vi "vision0.vi"(0 "Color Plane (Color Plane Extraction 1)":i32(ring)=2 items=["Red", "Green", "Blue", "Hue", "Saturation", "Luminance", "Value", "Intensity"], 1 "Range (Threshold 1)":cluster{"Lower value":sgl, "Upper value":sgl}={"Lower value"=199.0, "Upper value"=255.0}, 2 "Number of Erosion (Adv. Morphology 1)":i32=1, 3 "Square/Hexa (Square) (Adv. Morphology 1)":bool, 4 "Connectivity 4/8 (8) (Adv. Morphology 1)":bool=TRUE, 5 "Low Pass/High Pass (Low) (Adv. Morphology 1)":bool, 7 "error in":errorcluster) -> (20 "Number of Matches (Shape Matching 1)":i32, 21 "Shape Report (calibrated) (Shape Matching 1)":T2(array[cluster]) {"Score" format="%.2f"; "Centroid"."y" format="%.2f"; "Centroid"."x" format="%.2f"}, 22 "Centroid (Centroid 1)":cluster{"X Centroid":sgl, "Y Centroid":sgl} {"Y Centroid" format="%.2f"; "X Centroid" format="%.2f"}, 23 "Calibrated Centroid (Centroid 1)":cluster{"X Centroid":sgl, "Y Centroid":sgl} {"Y Centroid" format="%.2f"; "X Centroid" format="%.2f"}, 27 "error out":errorcluster)   [LabVIEW 2016]
uses:
  <vilib>/vision/NI_Vision_Development_Module.lvlib
panel:
  out "Image Out":T1(plugin-control)
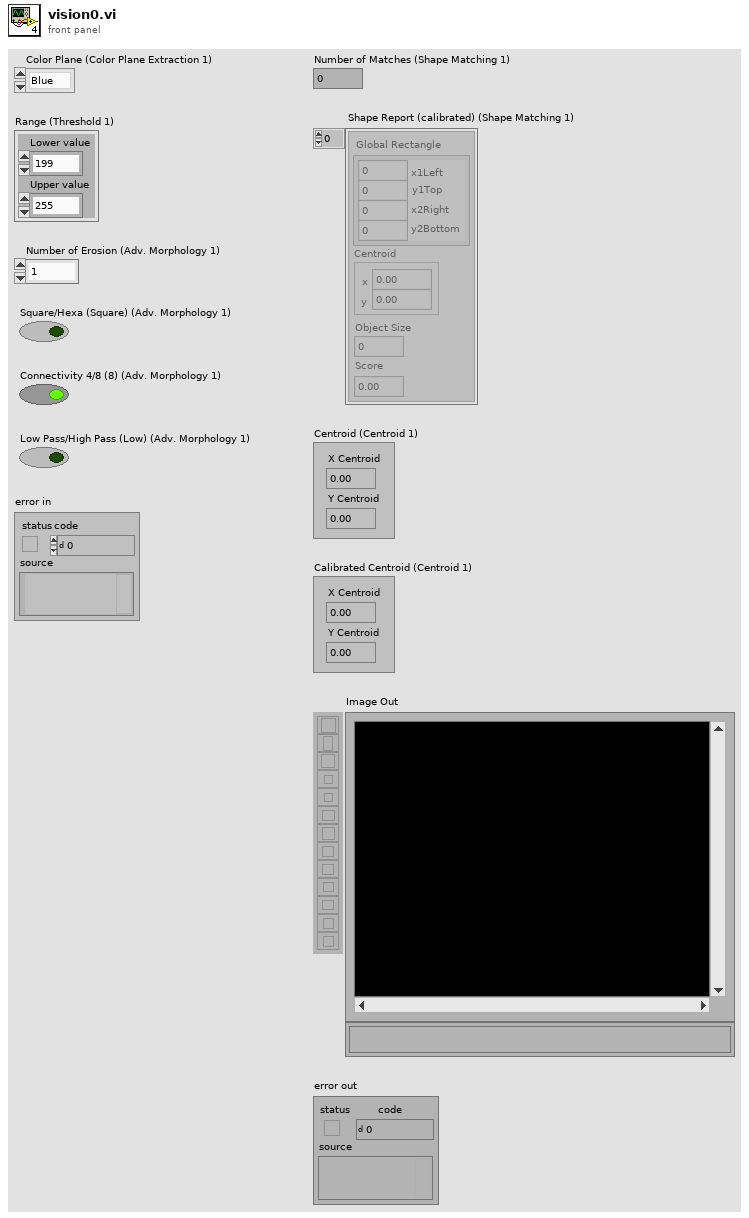
[diagram p1: front panel]
types:
  T1 = typedef "IMAQ Image.ctl" = refnum<image>
  T2 = cluster{"Global Rectangle":cluster{"x1Left":i32, "y1Top":i32, "x2Right":i32, "y2Bottom":i32}, "Centroid":cluster{"x":sgl, "y":sgl}, "Object Size":u32, "Score":dbl}[]
  T3 = typedef "Image Type" = u32
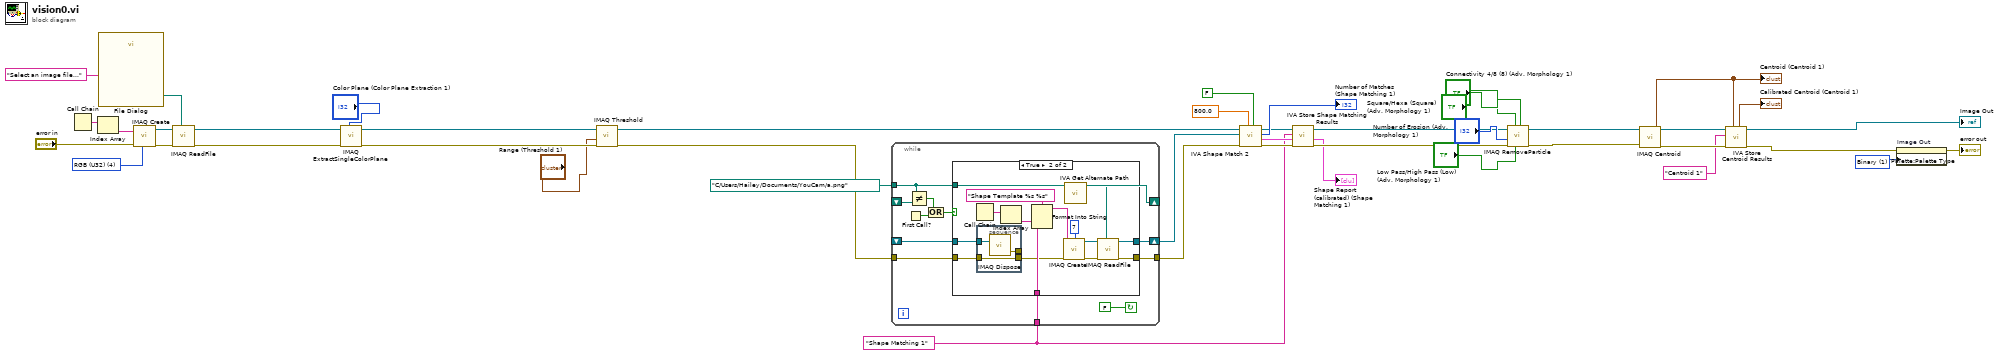
[diagram p0: block diagram]
diagram:
  w1 = u32 1 items=["Grayscale", "Binary", "Gradient", "Rainbow", "Temperature", "User Defined", "Binary 16 Bit", "Gradient 16 Bit", "Rainbow 16 Bit", "Temperature 16 Bit", "User Defined 16 Bit"] ("Palette Type")
  w16 = "Shape Matching 1" ("Step Name")
  w35 = T3 4 items=["Grayscale (U8)", "Grayscale (I16)", "Grayscale (SGL)", "Complex (CSG)", "RGB (U32)", "HSL (U32)", "RGB (U64)", "Grayscale (U16)"] ("Image Type")
  n1 = Call Chain() -> (call chain=w39:string[])
  n2 = Index Array(array=w39) -> (element=w38:string)  [unwired: 1 in]
  n3 = call "File Dialog"("prompt"="Select an image file...") -> ("selected path"=w36:path)  [unwired: 6 in, 8 out]
  n4 = call "IMAQ Create"("Image Name"=w38, "Image Type"=w35, "error in (no error)"="error in") -> ("New Image"=w42:T1, "error out"=w41:errorcluster)  [unwired: 1 in, 1 out]
  n5 = call "IMAQ ReadFile"("File Path"=w36, "error in (no error)"=w41, "Image"=w42) -> ("error out"=w43:errorcluster, "Image Out"=w33:T1)  [unwired: 2 in, 5 out]
  n6 = call "IMAQ ExtractSingleColorPlane"("Color Plane"="Color Plane (Color Plane Extraction 1)", "error in (no error)"=w43, "Image Src"=w33) -> ("error out"=w32:errorcluster, "Image Dst Out"=w30:T1)  [unwired: 1 in, 6 out]
  n7 = call "IMAQ Threshold"("error in (no error)"=w32, "Range"="Range (Threshold 1)", "Image Src"=w30) -> ("error out"=w29:errorcluster, "Image Dst Out"=w25:T1)  [unwired: 3 in, 4 out]
  n8 = while {
    shift-right: [w54] -> w17
    shift-left: _ -> [w53]
    tunnel: [w51] -> w18
    tunnel: w29 -> [w50]
    tunnel: path "C:/Users/Hailey/Documents/YouCam/a.png" ("Template Path") -> [w48]
    tunnel: w16 -> [w49]
    shift-right: [w48] -> _
    shift-left: _ -> [w47]
    stop <- FALSE continue-if-true
    n9 = First Call?() -> (First Call?: T/F=w46:bool)
    n10 = Not Equal?(x=w48, y=w47) -> (x != y?=w45:bool)
    n11 = Or(x=w45, y=w46) -> (x .or. y?=w44:bool)
    n12 = case shown="True" w44 {
      tunnel: [w56 w68] -> w54
      tunnel: w53 -> [w56 w59]
      tunnel: [w55 w66] -> w51
      tunnel: w50 -> [w55 w58]
      tunnel: w48 -> [_ w61]
      tunnel: w49 -> [_ w62]
      frame False {
      }
      frame True {
        n13 = Call Chain() -> (call chain=w64:string[])
        n14 = stacked-sequence {
          tunnel: w59 -> [w74]
          tunnel: w58 -> [w73]
          tunnel: [w73] -> w57
          tunnel: [w72] -> _
          frame #0 {
            n15 = call "IMAQ Dispose"("Image"=w74) -> ("error out"=w72:errorcluster)  [unwired: 2 in, 3 out]
          }
        }
        n16 = Index Array(array=w64) -> (element=w63:string)  [unwired: 1 in]
        n17 = Format Into String(format string="Shape Template %s %s" ("Image Name"), w63, w62) -> (resulting string=w71:string)  [unwired: 2 in, 1 out]
        n18 = call "IMAQ Create"("Border Size"=7, "Image Name"=w71, "error in (no error)"=w57) -> ("New Image"=w69:T1, "error out"=w67:errorcluster)  [unwired: 1 in, 1 out]
        n19 = call <vilib>:"IVA Get Alternate Path.vi"("Path In"=w61) -> ("Path Out"=w60:path)  [unwired: 10 out]
        n20 = call "IMAQ ReadFile"("File Path"=w60, "error in (no error)"=w67, "Image"=w69) -> ("error out"=w66:errorcluster, "Image Out"=w68:T1)  [unwired: 2 in, 5 out]
      }
    }
  }
  n21 = call <vilib>:"IVA Shape Match 2.vi"("Scale Invariance"=FALSE, "Minimal Score"=800.0, "error in (no error)"=w18, "Template"=w17, "Image Src"=w25) -> ("error out"=w24:errorcluster, "Shape Report"=w22:T2, "Number of Matches"=→"Number of Matches (Shape Matching 1)":i32, "Image Out"=w21:T1)  [unwired: 3 out]
  n22 = call <vilib>:"IVA Store Shape Matching Results.vi"("error in (no error)"=w24, "Shape Report"=w22, "Step Name"=w16, "Image in"=w21) -> ("error out"=w23:errorcluster, "Shape Report (calibrated)"=→"Shape Report (calibrated) (Shape Matching 1)":T2, "Image dup"=w11:T1)  [unwired: 5 out]
  n23 = call "IMAQ RemoveParticle"("Connectivity 4/8 (8)"="Connectivity 4/8 (8) (Adv. Morphology 1)", "Low Pass/High Pass (Low)"="Low Pass/High Pass (Low) (Adv. Morphology 1)", "Square/Hexa (Square)"="Square/Hexa (Square) (Adv. Morphology 1)", "error in (no error)"=w23, "Number of Erosion"="Number of Erosion (Adv. Morphology 1)", "Image Src"=w11) -> ("error out"=w10:errorcluster, "Image Dst Out"=w7:T1)  [unwired: 1 in, 3 out]
  n24 = call "IMAQ Centroid"("error in (no error)"=w10, "Image"=w7) -> ("error out"=w9:errorcluster, "Centroid"=w5:cluster{"X Centroid":sgl, "Y Centroid":sgl})  [unwired: 1 in, 1 out]
  "Centroid (Centroid 1)" <- w5
  n25 = call <vilib>:"IVA Store Centroid Results.vi"("Centroid in"=w5, "error in (no error)"=w9, "Step Name"="Centroid 1", "Image in"=w7) -> ("error out"=w8:errorcluster, "Image dup"=→"Image Out":T1, "Calibrated Centroid"=→"Calibrated Centroid (Centroid 1)":cluster{"X":sgl, "Y":sgl})  [unwired: 5 out]
  n26 = property on="Image Out" class="ImageControl"(error in=w8, "Palette:Palette Type"=w1) -> (error out=→"error out":errorcluster)  [unwired: 1 in, 1 out]
